vi "Outputs SW Set.vi"(7 "Current Time":timestamp format="%<%x %.3X>T", 8 "HW Config":T1={"ExtendHW Ver"=0, "CAN"={"ID"=0, "Bus"=""}, "Output"={"Inverted"=FALSE, "Neutral"=enum."Override to Coast", "Max"={"FWD"=1.0, "REV"=-1.0}, "Min"={"FWD"=0.0, "REV"=0.0}, "OL Ramp Rate (S)"=0.0, "Dead Band"=0.0, "CL Ramp Rate (S)"=0.0}, "CL"={"Gains"={"P"=1.0, "I"=0.01, "D"=0.0, "F"=0.0}, "Error Allowed"={"High"=0.0, "Low"=0.0}, "I Zone"={"High"=10000.0, "Low"=-1000.0}, "Max Out"={"FWD"=1.0, "REV"=-1.0}, "Max I Accu"={"High"=10.0, "Low"=-10.0}, "CL Ramp Rate (S)"=0.0}, "MM"={"Cruise Velocity"=5000, "Acceleration"=5000}, "TravelLimits"={"Hard"={"FWD Switch Normal"=enum."Normally Open", "FWD On will Zero Encoder "=FALSE, "REV Switch Normal"=enum."Normally Open", "REV On will Zero Encoder "=FALSE}, "Soft"={"FWD"={"Enable"=FALSE, "Counts"=0}, "REV"={"Enable"=FALSE, "Counts"=0}}}, "StatorLimit"={"Enable"=FALSE, "Current Limit"=0.0, "Threshold Current"=0.0, "Threshold Time"=0.0}, "Cancoder"={"ID"=0, "CW(t) CCW(f)"=TRUE, "Zero Offset"=0.0}} {"TravelLimits"."Soft"."REV"."Counts" format="%#.0f"; "TravelLimits"."Soft"."FWD"."Counts" format="%#.0f"; "Output"."Min"."REV" format="%.2f"; "Output"."Min"."FWD" format="%.2f"; "Output"."Max"."REV" format="%.2f"; "Output"."Max"."FWD" format="%.2f"; "CL"."Max I Accu"."Low" format="%#.8f"; "CL"."Max I Accu"."High" format="%#.8f"; "CL"."Gains"."F" format="%#.8f"; "CL"."Gains"."D" format="%#.8f"; "CL"."Gains"."I" format="%#.8f"; "CL"."Gains"."P" format="%#.8f"; "CL"."Error Allowed"."Low" format="%#.8f"; "CL"."Error Allowed"."High" format="%#.8f"; "CL"."I Zone"."Low" format="%#.8f"; "CL"."I Zone"."High" format="%#.8f"; "CL"."Max Out"."REV" format="%.2f"; "CL"."Max Out"."FWD" format="%.2f"}, 9 "SW Config":T17={"ExtendSW Ver"=0, "Home Speed (0-1)"=0.2, "Enable Current Limit On Homing"=FALSE, "At Position Delay(S)"=0.2}, 10 "Sensor Values":T19, 11 "SW Output":T18) -> (3 "SW Output Out":T18)   [LabVIEW 2020]
uses:
  Shared Code/TypeDefs/Cluster_FX CloseLoop Values.ctl
  Shared Code/TypeDefs/Cluster_FX Limit Switchs.ctl
  Shared Code/TypeDefs/Cluster_FX Current Values.ctl
  Shared Code/TypeDefs/Cluster_FWD  REV Values.ctl
  Shared Code/TypeDefs/Cluster_High-Low.ctl
  Shared Code/TypeDefs/Cluster_PID Gains.ctl
  Shared Code/TypeDefs/Cluster_SRX SLOT PID Config.ctl
  Shared Code/TypeDefs/Cluster_SRX Motion Magic Parameters.ctl
  Shared Code/TypeDefs/Cluser_CAN Data.ctl
  <vilib>/Rock Robotics/WPI/ThirdParty/Phoenix-LabVIEW/Motor Controller/Controls/CTRE_Phoenix_MotorControl_NeutralMode.ctl
  Shared Code/TypeDefs/Cluster_Config SRX Motor Output.ctl
  <vilib>/Rock Robotics/WPI/ThirdParty/Phoenix-LabVIEW/Motor Controller/Controls/CTRE_Phoenix_MotorControl_LimitSwitchNormal.ctl
  Shared Code/TypeDefs/Cluser_Hard Limits.ctl
  Shared Code/TypeDefs/Cluser_Enable-Value I32.ctl
  Shared Code/TypeDefs/Cluser_Config_Soft Limits.ctl
  Shared Code/TypeDefs/Cluser_Limit Travel Config.ctl
  Shared Code/TypeDefs/Cluster_Extend_SW Output Data.ctl
  Shared Code/TypeDefs/Cluster_FX Integrated Sensor Values.ctl
  Shared Code/TypeDefs/Cluster_Extend HW Outputs.ctl
  Shared Code/TypeDefs/Cluster_Extend_Config SW Values.ctl
  Shared Code/TypeDefs/Cluser_Config_Current Limits.ctl
  Shared Code/TypeDefs/Cluster_Extend_Config HW Values.ctl
  Shared Code/TypeDefs/Cluster_FX Sensor Values.ctl
  Shared Code/TypeDefs/Cluster_Cancoder_Config Data.ctl
panel:
  # "Tune Output\nto 1023 Max"
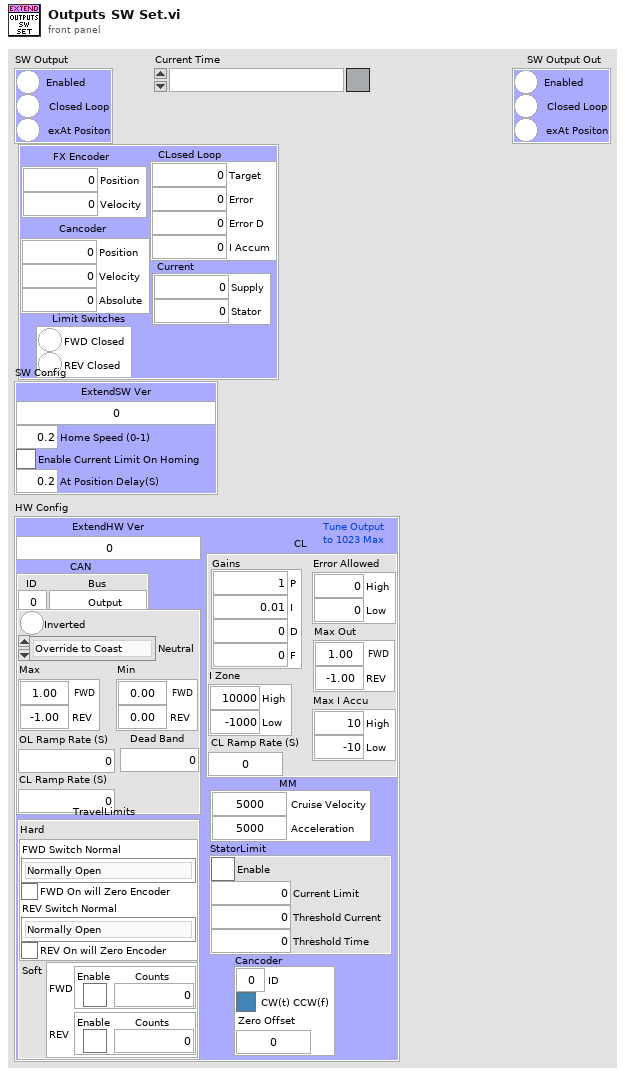
[diagram p1: front panel]
types:
  T1 = typedef "Cluster_Extend_Config HW Values.ctl" = cluster{"ExtendHW Ver":u64, "CAN":T2, "Output":T3, "CL":T6, "MM":T9, "TravelLimits":T10, "StatorLimit":T15, "Cancoder":T16}
  T2 = typedef "Cluser_CAN Data.ctl" = cluster{"ID":u8, "Bus":string}
  T3 = typedef "Cluster_Config SRX Motor Output.ctl" = cluster{"Inverted":bool, "Neutral":T4, "Max":T5, "Min":T5, "OL Ramp Rate (S)":dbl, "Dead Band":dbl, "CL Ramp Rate (S)":dbl}
  T4 = typedef "CTRE_Phoenix_MotorControl_NeutralMode.ctl" = enum8{"EEPROMSetting", "Override to Coast", "Override to Brake"}
  T5 = typedef "Cluster_FWD  REV Values.ctl" = cluster{"FWD":dbl, "REV":dbl}
  T6 = typedef "Cluster_PID Config.ctl" = cluster{"Gains":T7, "Error Allowed":T8, "I Zone":T8, "Max Out":T5, "Max I Accu":T8, "CL Ramp Rate (S)":dbl}
  T7 = typedef "Cluster_PID Gains.ctl" = cluster{"P":dbl, "I":dbl, "D":dbl, "F":dbl}
  T8 = typedef "Cluster_High-Low.ctl" = cluster{"High":dbl, "Low":dbl}
  T9 = typedef "Cluster_SRX Motion Magic Parameters.ctl" = cluster{"Cruise Velocity":i32, "Acceleration":i32}
  T10 = typedef "Cluser_Limit Travel Config.ctl" = cluster{"Hard":T11, "Soft":T13}
  T11 = typedef "Cluser_Hard Limits.ctl" = cluster{"FWD Switch Normal":T12, "FWD On will Zero Encoder ":bool, "REV Switch Normal":T12, "REV On will Zero Encoder ":bool}
  T12 = typedef "CTRE_Phoenix_MotorControl_LimitSwitchNormal.ctl" = enum16{"Normally Open", "Normally Closed", "Disabled"}
  T13 = typedef "Cluser_Config_Soft Limits.ctl" = cluster{"FWD":T14, "REV":T14}
  T14 = typedef "Cluser_Enable-Value I32.ctl" = cluster{"Enable":bool, "Counts":i32}
  T15 = typedef "Cluser_Config_Current Limits.ctl" = cluster{"Enable":bool, "Current Limit":dbl, "Threshold Current":dbl, "Threshold Time":dbl}
  T16 = typedef "Cluster_Cancoder_Config Data.ctl" = cluster{"ID":u8, "CW(t) CCW(f)":bool, "Zero Offset":dbl}
  T17 = typedef "Cluster_Extend_Config SW Values.ctl" = cluster{"ExtendSW Ver":u64, "Home Speed (0-1)":dbl, "Enable Current Limit On Homing":bool, "At Position Delay(S)":dbl}
  T18 = typedef "Cluster_Extend_SW Output Data.ctl" = cluster{"Enabled":bool, "Closed Loop":bool, "exAt Positon":bool}
  T19 = typedef "Cluster_Extend HW Outputs.ctl" = cluster{"CLosed Loop":T20, "Limit Switches":T21, "Current":T22, "FX Encoder":T23, "Cancoder":T24}
  T20 = typedef "Cluster_FX CloseLoop Values.ctl" = cluster{"Target":dbl, "Error":i32, "Error D":dbl, "I Accum":dbl}
  T21 = typedef "Cluster_FX Limit Switchs.ctl" = cluster{"FWD Closed":bool, "REV Closed":bool}
  T22 = typedef "Cluster_FX Current Values.ctl" = cluster{"Supply":dbl, "Stator":dbl}
  T23 = typedef "Cluster_FX Sensor Values.ctl" = cluster{"Position":i32, "Velocity":i32}
  T24 = typedef "Cluster_FX Integrated Sensor Values.ctl" = cluster{"Position":dbl, "Velocity":dbl, "Absolute":dbl}
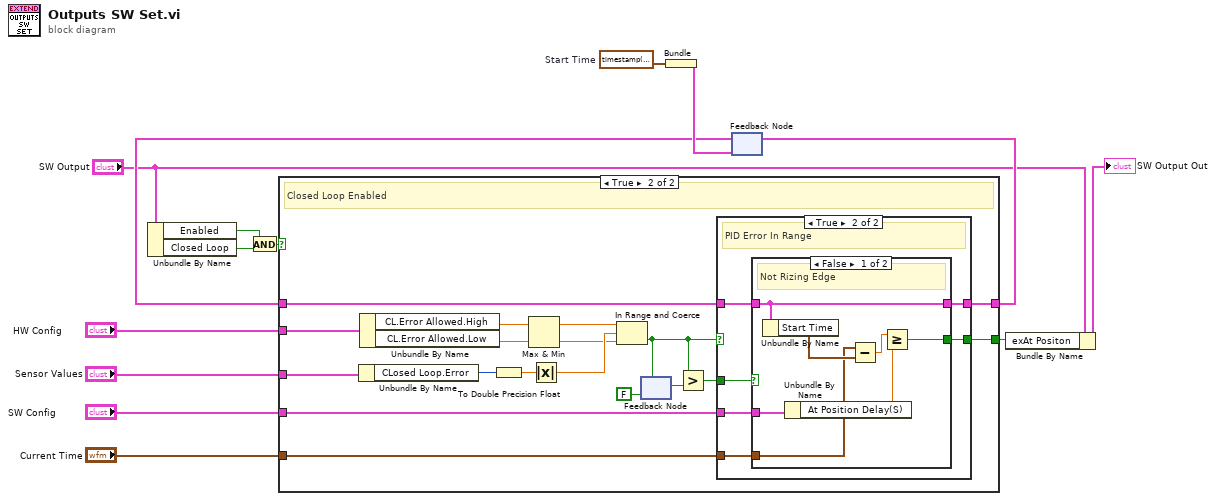
[diagram p0: block diagram]
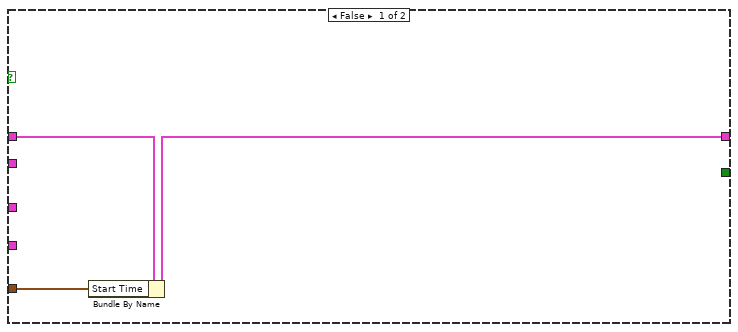
[diagram p2: hidden frame]
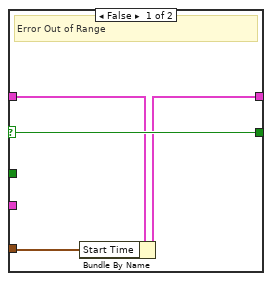
[diagram p3: hidden frame]
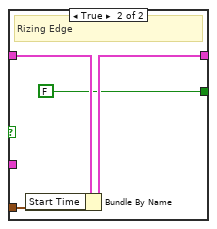
[diagram p4: hidden frame]
diagram:
  w8 = timestamp(0 s since 1904-01-01)  # Start Time
  n1 = Unbundle By Name("SW Output") -> ("Enabled"=w14:bool, "Closed Loop"=w13:bool)
  n2 = And(x=w14, y=w13) -> (x .and. y?=w9:bool)
  n3 = Bundle("Start Time"=w8) -> (w7:cluster{"Start Time":timestamp})  [unwired: 1 in]
  n4 = feedback #1(w7) -> (w6:cluster{"Start Time":timestamp})
  n5 = case shown="True" w9 {
    tunnel: "SW Config" -> [_ w35]
    tunnel: "Sensor Values" -> [_ w33]
    tunnel: "Current Time" -> [w16 w24]
    tunnel: w6 -> [w17 w34]
    tunnel: [w15 w25] -> w5
    tunnel: [_ w23] -> w1
    tunnel: "HW Config" -> [_ w32]
    frame False {
      n6 = Bundle By Name(cluster=w17, "Start Time"=w16) -> (w15:cluster{"Start Time":timestamp})
    }
    frame True {
      # "Closed Loop Enabled"
      n7 = Unbundle By Name(w33) -> ("CLosed Loop.Error"=w31:i32)
      n8 = Unbundle By Name(w32) -> ("CL.Error Allowed.High"=w19:dbl, "CL.Error Allowed.Low"=w21:dbl)
      n9 = To Double Precision Float(number=w31) -> (double precision float=w30:dbl)
      n10 = Max & Min(x=w19, y=w21) -> (max(x,y)=w18:dbl, min(x,y)=w20:dbl)
      n11 = Absolute Value(x=w30) -> (abs(x)=w22:dbl)
      n12 = In Range and Coerce(upper limit=w18, x=w22, lower limit=w20) -> (In Range?=w27:bool)  [unwired: 1 out]
      n13 = feedback #2(FALSE) -> (w29:bool)
      n14 = feedback-in #2(w27) -> ()
      n15 = Greater?(x=w27, y=w29) -> (0:w26:bool)
      n16 = case shown="True" w27 {
        selector: w27 -> [w39 _]
        tunnel: w35 -> [_ w45]
        tunnel: w34 -> [w36 w43]
        tunnel: w26 -> [_ w44]
        tunnel: [w37 w42] -> w25
        tunnel: w24 -> [w38 w41]
        tunnel: [w39 w40] -> w23
        frame False {
          # "Error Out of Range"
          n17 = Bundle By Name(cluster=w36, "Start Time"=w38) -> (w37:cluster{"Start Time":timestamp})
        }
        frame True {
          # "PID Error In Range"
          n18 = case shown="False" w44 {
            tunnel: w45 -> [w48 _]
            tunnel: w43 -> [w52 w54]
            tunnel: [w52 w55] -> w42
            tunnel: w41 -> [w50 w56]
            tunnel: [w46 FALSE] -> w40
            frame False {
              # "Not Rizing Edge"
              n19 = Unbundle By Name(w52) -> ("Start Time"=w51:timestamp)
              n20 = Unbundle By Name(w48) -> ("At Position Delay(S)"=w47:dbl)
              n21 = Subtract(x=w50, y=w51) -> (x-y=w49:dbl)
              n22 = Greater Or Equal?(x=w49, y=w47) -> (x >= y?=w46:bool)
            }
            frame True {
              # "Rizing Edge"
              n23 = Bundle By Name(cluster=w54, "Start Time"=w56) -> (w55:cluster{"Start Time":timestamp})
            }
          }
        }
      }
    }
  }
  n24 = feedback-in #1(w5) -> ()
  n25 = Bundle By Name(cluster="SW Output", "exAt Positon"=w1) -> (→"SW Output Out":T18)
